vi "time_sql_test.vi"() -> ()   [LabVIEW 2017]
uses:
  <vilib>/addons/database/Connection.llb/DB Tools Open Connec (Path).vi
  <userlib>/_OpenG.lib/array/array.llb/Remove Duplicates from 1D Array (String)__ogtk.vi
  <vilib>/addons/database/NI_Database_API.lvlib
panel:
  out "x-y":timestamp
  out "resulting string":string
  in  "Get Backup\nTreshold Time":timestamp caption="Get Backup Treshold Time"
  out "Output Array":variant[](array[variant])
  out "data":string[][](array[string])
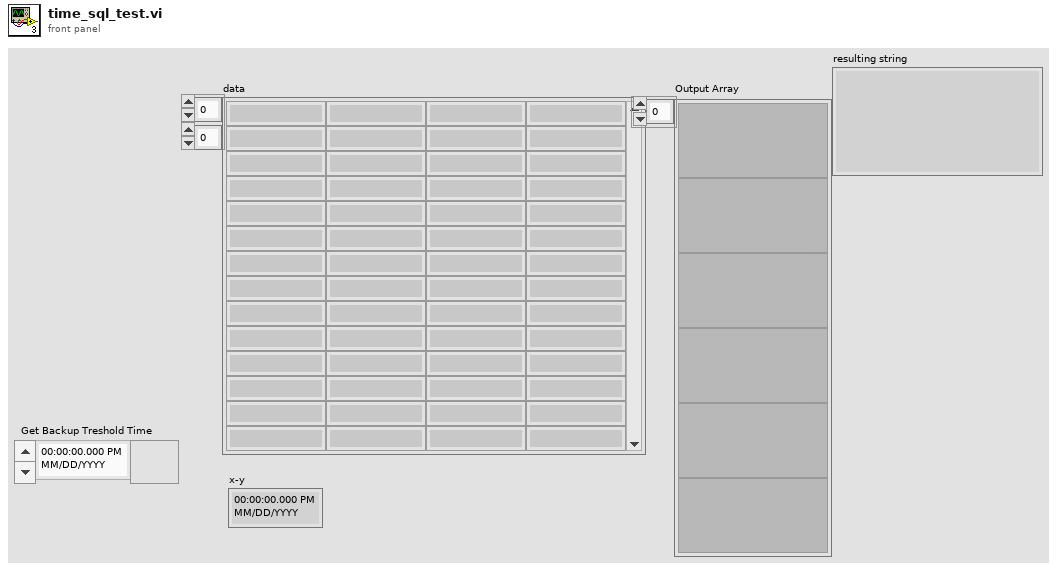
[diagram p1: front panel]
types:
  T1 = typedef "LVDateTimeRec.ctl" = cluster{"fractional second":dbl, "second":i32, "minute":i32, "hour":i32, "day of month":i32, "month":i32, "year":i32, "day of week":i32, "day of year":i32, "DST":i32}
  T2 = typedef "NI_Database_API.lvlib/Conn ObjectReference.ctl" = refnum<k1>
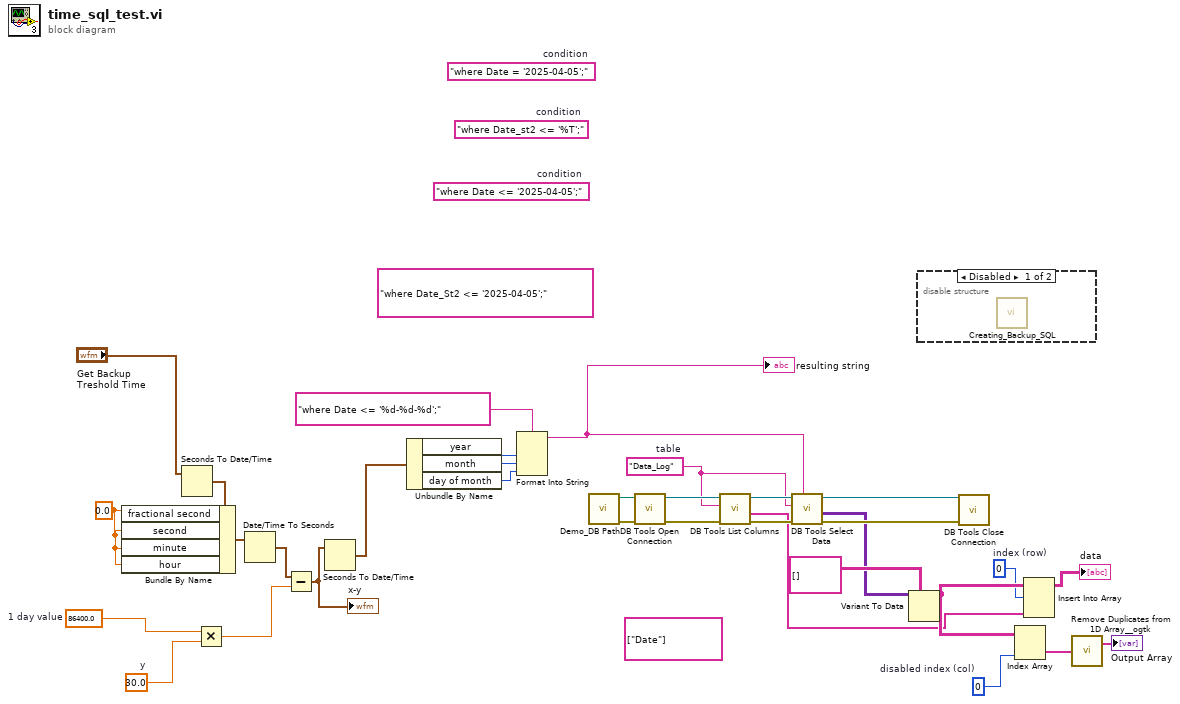
[diagram p0: block diagram]
diagram:
  w5 = 0.0 ("fractional second")
  w8 = 0  # index (row)
  w12 = 30.0  # y
  w13 = 86400.0  # 1 day value
  w14 = 0  # disabled index (col)
  (unwired) string[] ["Date"] ("format string")
  (unwired) "where Date_St2 <= '2025-04-05';" ("format string")
  (unwired) "where Date_st2 <= '%T';"  # condition
  (unwired) "where Date = '2025-04-05';"  # condition
  (unwired) "where Date <= '2025-04-05';"  # condition
  w25 = "Data_Log"  # table
  n1 = Seconds To Date/Time(time stamp (now)="Get Backup\nTreshold Time") -> (date time rec=w6:T1)  [unwired: 1 in]
  n2 = Bundle By Name(cluster=w6, "fractional second"=w5, "second"=w5, "minute"=w5, "hour"=w5) -> (w7:T1)
  n3 = Multiply(x=w13, y=w12) -> (x*y=w3:dbl)
  n4 = Date/Time To Seconds(2:w7) -> (0:w2:timestamp)  [unwired: 1 in]
  n5 = Subtract(x=w2, y=w3) -> (x-y=w1:timestamp)
  "x-y" <- w1
  n6 = Seconds To Date/Time(time stamp (now)=w1) -> (date time rec=w20:T1)  [unwired: 1 in]
  n7 = Unbundle By Name(w20) -> ("year"=w19:i32, "month"=w18:i32, "day of month"=w17:i32)
  n8 = Format Into String(format string="where Date <= '%d-%d-%d';", w19, w18, w17) -> (resulting string=w16:string)  [unwired: 2 in, 1 out]
  "resulting string" <- w16
  n9 = call "Demo_DB Path.vi"() -> ("error out"=w33:errorcluster, "DB Path"=w32:path)  [unwired: 10 in]
  n10 = call-poly <vilib>:"DB Tools Open Connection.vi"("error in (no error)"=w33, "connection information"=w32) -> ("error out"=w29:errorcluster, "connection reference"=w27:T2)  [unwired: 6 in]
  n11 = call <vilib>:"DB Tools List Columns.vi"("error in (no error)"=w29, "table"=w25, "connection reference"=w27) -> ("error out"=w28:errorcluster, "columns"=w9:string[], "connection reference out"=w26:T2)  [unwired: 1 in, 1 out]
  n12 = call <vilib>:"DB Tools Select Data.vi"("condition"=w16, "error in (no error)"=w28, "table"=w25, "connection reference"=w26) -> ("error out"=w31:errorcluster, "data"=w23:variant[][], "connection reference out"=w30:T2)  [unwired: 2 in]
  n13 = Variant To Data(type=string[][] [], Variant=w23) -> (data=w11:string[][])  [unwired: 1 in, 1 out]
  n14 = disable-structure shown="Disabled" {
    frame Disabled {
      n15 = call "Creating_Backup_SQL.vi"() -> ()  [unwired: 9 in, 3 out]
    }
    frame Enabled {
    }
  }
  n16 = call <vilib>:"DB Tools Close Connection.vi"("error in (no error)"=w31, "connection reference"=w30) -> ()  [unwired: 5 in, 1 out]
  n17 = Index Array(array=w11, index (col)=w14) -> (element=w15:string[])  [unwired: 1 in]
  n18 = Insert Into Array(array=w11, index (row)=w8, new element=w9) -> (→"data":string[][])  [unwired: 1 in]
  n19 = call-poly <userlib>:"Remove Duplicates from 1D Array__ogtk.vi"("Input Array"=w15) -> ("Output Array"=→"Output Array":string[])  [unwired: 1 out]
